vi "Parse MREU Variant.vi"(10 "Variant":variant) -> (2 "MREU Telemetry":T1 {"DSCR"."Raw_DSCR" format="%04x"; "DSCR"."DM_EE_ERRADD"."MSW" format="%02x"; "DSCR"."DM_EE_ERRADD"."LSW" format="%04x"; "DSCR"."DSCR_5"."DM_INTVL" format="%03x"; "DSCR"."TMR_30_31"."TMR1_CNT" format="%1x"; "DSCR"."TMR_30_31"."TMR0_CNT" format="%1x"; "DSCR"."TMR_26_27"."TMR1_CNT" format="%1x"; "DSCR"."TMR_26_27"."TMR0_CNT" format="%1x"; "DSCR"."TMR_24_25"."TMR1_CNT" format="%1x"; "DSCR"."TMR_24_25"."TMR0_CNT" format="%1x"; "DSCR"."TMR_28_29"."TMR1_CNT" format="%1x"; "DSCR"."TMR_28_29"."TMR0_CNT" format="%1x"; "DSCR"."TMR_16_17"."TMR1_CNT" format="%1x"; "DSCR"."TMR_16_17"."TMR0_CNT" format="%1x"; "DSCR"."TMR_22_23"."TMR1_CNT" format="%1x"; "DSCR"."TMR_22_23"."TMR0_CNT" format="%1x"; "DSCR"."TMR_20_21"."TMR1_CNT" format="%1x"; "DSCR"."TMR_20_21"."TMR0_CNT" format="%1x"; "DSCR"."TMR_18_19"."TMR1_CNT" format="%1x"; "DSCR"."TMR_18_19"."TMR0_CNT" format="%1x"; "DSCR"."TMR_14_15"."TMR1_CNT" format="%1x"; "DSCR"."TMR_14_15"."TMR0_CNT" format="%1x"; "DSCR"."TMR_12_13"."TMR1_CNT" format="%1x"; "DSCR"."TMR_12_13"."TMR0_CNT" format="%1x"; "DSCR"."TMR_10_11"."TMR1_CNT" format="%1x"; "DSCR"."TMR_10_11"."TMR0_CNT" format="%1x"; "DSCR"."TMR_8_9"."TMR1_CNT" format="%1x"; "DSCR"."TMR_8_9"."TMR0_CNT" format="%1x"; "DSCR"."TMR_6_7"."TMR1_CNT" format="%1x"; "DSCR"."TMR_6_7"."TMR0_CNT" format="%1x"; "DSCR"."TMR_4_5"."TMR1_CNT" format="%1x"; "DSCR"."TMR_4_5"."TMR0_CNT" format="%1x"; "DSCR"."TMR_2_3"."TMR1_CNT" format="%1x"; "DSCR"."TMR_2_3"."TMR0_CNT" format="%1x"; "DSCR"."TMR_0_1"."TMR1_CNT" format="%1x"; "DSCR"."TMR_0_1"."TMR0_CNT" format="%1x"; "Full ESCR"."RawESCR" format="%04x"; "Full ESCR"."RTR2"."Value" format="%04x"; "Full ESCR"."CLK_DRFT"."Value" format="%04x"; "Full ESCR"."CLK_ADJ"."Value" format="%04x"; "Full ESCR"."MT_ERRADD"."Value" format="%04x"; "Full ESCR"."TC_ERRADD"."Value" format="%04x"; "Full ESCR"."Device_ID"."Value" format="%04x"; "Full ESCR"."SCT"."SCT" format="%04x"; "Full ESCR"."SCT"."RTI" format="%02x"; "Full ESCR"."DMA_ERRADD"."LSW" format="%04x"; "Full ESCR"."DMA_ERRADD"."MSW" format="%02x"; "Full ESCR"."EEPROM_ERRADD"."LSW" format="%04x"; "Full ESCR"."EEPROM_ERRADD"."MSW" format="%02x"; "Full ESCR"."SCR_ERRADD"."LSW" format="%04x"; "Full ESCR"."SCR_ERRADD"."MSW" format="%02x"; "Full_PM"."RawPM" format="%04x"; "Full_PM"."CKSUM"."Value" format="%04x"; "Full_PM"."BUALM_SNZ"."LSW" format="%04x"; "Full_PM"."BUALM_SNZ"."MSW" format="%02x"; "Full_PM"."BUALM"."LSW" format="%04x"; "Full_PM"."BUALM"."MSW" format="%02x"; "Full_PM"."PALM_SNZ"."LSW" format="%04x"; "Full_PM"."PALM_SNZ"."MSW" format="%02x"; "Full_PM"."PALM"."LSW" format="%04x"; "Full_PM"."PALM"."MSW" format="%02x"; "Full_PM"."MissionClock"."Val_19_4" format="%04x"; "Full_PM"."MissionClock"."Val_35_20" format="%04x"; "Full_PM"."MissionClock"."Val_51_36" format="%04x"; "Full_PM"."FP_WDT"."Value" format="%04x"; "Full DISC"."RawDiscIn" format="%04x"; "Full DISC"."RawDISC" format="%04x"})   [LabVIEW 2019]
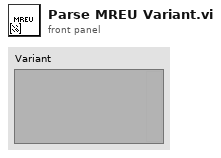
[diagram p1: front panel]
types:
  T1 = cluster{"NoResponse":bool, "Analog Telemetry":waveform(dbl)[], "Full ESCR":cluster{"ESCR 7":cluster{"RT_TC_ERAD_WR":bool, "SCR_ERAD_WR":bool, "EE_ERAD_WR":bool, "DMA_ERAD_WR":bool, "CLKADJ_WR":bool, "CLKDRFT_WR":bool, "MT_ERAD_WR":bool, "BUS_CONF_INH":bool, "VMON_OVRD":bool, "VMN_OVRD_CTL":bool, "PM_TEST_EN":bool, "VMON_P3V":bool, "VMON_P5V":bool, "VMON_N12V":bool, "VMON_P12V":bool, "SET_CLRn":bool}, "ESCR 6":cluster{"DMA_DBE":bool, "DMA_SBE":bool, "UNUSED":bool, "ILL_MEM_ACC":bool, "EE_RD_URUN":bool, "EE_WR_ORUN":bool, "EE_WR_TIMEOUT":bool, "EE_WR_BUSY":bool, "BANK_0_WPV":bool, "BANK_1_WPV":bool, "BANK_2_WPV":bool, "BANK_3_WPV":bool, "FSW_HIMEM_WPV":bool, "FSW_BNK_WPV":bool, "DMA_SRAM_WPV":bool, "SET_CLRn":bool}, "ESCR 5":cluster{"EEPROM_DBE":bool, "EEPROM_SBE":bool, "AI_MOVE_CONF":bool, "DEF_BANK_ERR":bool, "PREEMPTION":bool, "UNEX_OPCODE":bool, "ILLEGAL_OPCOD":bool, "RANGE_ERR":bool, "RSB_ABORT":bool, "TLM_ADDR_CFG":bool, "RZ_EN":bool, "TLM_DATA_ERR":bool, "TLM_TIME_OUT":bool, "TLM_FR_ERR":bool, "TLM_PAR_ERR":bool, "SET_CLRn ":bool}, "ESCR_4":cluster{"ACT_BANK_0":bool, "ACT_BANK_1":bool, "EXT_DEF_BANK_0":bool, "EXT_DEF_BANK_1":bool, "FSW_DEF_BANK_0":bool, "FSW_DEF_BANK_1":bool, "DEF_BANKSEL_0":bool, "DEF_BANKSEL_1":bool, "WP_BNK0_INH":bool, "WP_BNK1_INH":bool, "WP_BNK2_INH":bool, "WP_BNK3_INH":bool, "WP_HIME_INH":bool, "ILL_BNK_CHNG":bool, "WP_SRAM_INH":bool, "SET_CLRn ":bool}, "ESCR 3":cluster{"SCR_DBE":bool, "SCR_SBE":bool, "UNUSED[2]":bool, "UNUSED[3]":bool, "UNUSED[4]":bool, "UNUSED[5]":bool, "SRAM_SCR_EN":bool, "PROM_SCR_EN":bool, "BRG_MOD_0":bool, "BRG_MOD_1":bool, "BRG_MOD_2":bool, "PM_CKSUM_EN":bool, "UNUSED[12]":bool, "UNUSED[13] ":bool, "UNUSED[14]":bool, "SET_CLRn":bool}, "ESCR 2":cluster{"CH_DIS_B":bool, "UNUSED[1]":bool, "LVDS_SCF_B":bool, "RT_SCF_B":bool, "BRG_SCF_B":bool, "BUS_CONF_B":bool, "BR_POW_ON":bool, "BR_POW_EN":bool, "CH_DIS_A":bool, "UNUSED[9]":bool, "LVDS_SCF":bool, "RT_SCF":bool, "BRG_SCF_A":bool, "BUS_CONF_A":bool, "BIDI_EN":bool, "SET_CLRn":bool}, "ESCR 1":cluster{"TC_DBE":bool, "TC_SBE":bool, "RTI_ORUN":bool, "MT_PRG_ERR":bool, "HCR_ERR":bool, "RT_DBE":bool, "RT_SBE":bool, "EDAC_EN":bool, "AZEN":bool, "TC_RUN":bool, "COLD_START":bool, "SSYSF_EXT":bool, "RTI_FREQ_0":bool, "RTI_FREQ_1":bool, "SSYSF_INT":bool, "SET_CLRn":bool}, "CLK_DRFT":cluster{"Value":u16}, "CLK_ADJ":cluster{"Value":u16}, "MT_ERRADD":cluster{"Value":u16}, "TC_ERRADD":cluster{"Value":u16}, "Device_ID":cluster{"Value":u16}, "Board_ID":cluster{"ID":u16, "Board Type":enum16{"BB", "EM_SKT", "EM_AX2K", "EM_RTAX", "FM_SKT", "FM_RTAX"}}, "SCT":cluster{"SCT":u16, "RTI":u8}, "DMA_ERRADD":cluster{"LSW":u16, "MSW":u8}, "EEPROM_ERRADD":cluster{"LSW":u16, "MSW":u8}, "SCR_ERRADD":cluster{"LSW":u16, "MSW":u8}, "RTR2":cluster{"Value":u16}, "RawESCR":u16[]}, "Full_PM":cluster{"CKSUM":cluster{"Value":u16}, "PWR_LDSHD":cluster{"LOADSHED_PWR_L":bool, "LOADSHED_PWR_H":bool, "UNUSED[2]":bool, "UNUSED[3]":bool, "UNUSED[4]":bool, "UNUSED[5]":bool, "UNUSED[6]":bool, "UNUSED[7]":bool, "LOADSHEDL_EN":bool, "LOADSHEDH_EN":bool, "XSWU_OUT_MSK":bool, "UNUSED[11]":bool, "UNUSED[12]":bool, "UNUSED[13]":bool, "UNUSED[14]":bool, "SET_CLRn":bool}, "FPWDG_STAT":cluster{"UNUSED[0]":bool, "UNUSED[1]":bool, "UNUSED[2]":bool, "UNUSED[3]":bool, "UNUSED[4]":bool, "UNUSED[5]":bool, "UNUSED[6]":bool, "UNUSED[7]":bool, "UNUSED[8]":bool, "UNUSED[9]":bool, "FPWDG_INH":bool, "FPWDG_INH0":bool, "FPWDG_INH1":bool, "FPWDG_INH2":bool, "FPWDG_EXP":bool, "UNUSED[15]":bool}, "PWR_STAT":cluster{"POR1_EVT":bool, "POR2_EVT":bool, "PALM_EXP_EVT":bool, "XSWU_IN_EVT":bool, "USER1_EVT":bool, "USER2_EVT":bool, "GSE_EVT":bool, "POWER_POS_EVT":bool, "BOI_EVT":bool, "BUALM_EXP_EVT":bool, "UV_TRIP_EVT":bool, "MCLOCK_0":bool, "MCLOCK_1":bool, "MCLOCK_2":bool, "MCLOCK_3":bool, "SET_CLRn":bool}, "PWR_MSK":cluster{"UNUSED[0]":bool, "POR2_MSK":bool, "PALM_EXP_MSK":bool, "XSWU_IN_MSK":bool, "USER1_MSK":bool, "USER2_MSK":bool, "GSE_MSK":bool, "PWR_POS_MSK":bool, "BOI_MSK":bool, "BUALM_EXP_MSK":bool, "UV_TRIP_MSK":bool, "UNUSED[11]":bool, "BUALM_STEER":bool, "SELFCHK_MSK":bool, "CHKSUM_FAIL":bool, "SET_CLRn":bool}, "PWR_ACK":cluster{"COLD_START":bool, "POR2_WU":bool, "PALM_EXP_WU":bool, "XSWU_IN_WU":bool, "USER1_WU":bool, "USER2_WU":bool, "GSE_WU":bool, "POWER_POS_WU":bool, "BOI":bool, "BUALM_EXP":bool, "UV_TRIP":bool, "NAPPED":bool, "BUALM_EXP_WU":bool, "SELFCHK_FAIL":bool, "SLEEP_PNDG":bool, "SET_CLRn":bool}, "PWR_CTRL":cluster{"PWR_EN":bool, "PALM_VALID":bool, "PALM_SNZ_VALID":bool, "BUALM_VALID":bool, "BUALM_SNZ_VALID":bool, "MC_VALID":bool, "UNUSED[6]":bool, "FSM_BIT":bool, "Prev_State":enum16{"Sleep_00", "Deadman_01", "Awake_10", "Nap_11"}, "Curr_State":enum16{"Sleep_00", "Deadman_01", "Awake_10", "Nap_11"}, "POWER_POS":bool, "UNUSED[13]":bool, "UNUSED[14]":bool, "SET_CLRn":bool}, "BUALM_SNZ":cluster{"LSW":u16, "MSW":u8}, "BUALM":cluster{"LSW":u16, "MSW":u8}, "PALM_SNZ":cluster{"LSW":u16, "MSW":u8}, "PALM":cluster{"LSW":u16, "MSW":u8}, "MissionClock":cluster{"Val_19_4":u16, "Val_35_20":u16, "Val_51_36":u16}, "FP_WDT":cluster{"Value":u16}, "PWR_OFF_EN":cluster{"PWR_OFF_L_0":bool, "PWR_OFF_H_0":bool, "PWR_OFF_L_1":bool, "PWR_OFF_H_1":bool, "PWR_OFF_L_2":bool, "PWR_OFF_H_2":bool, "PWR_OFF_L_3":bool, "PWR_OFF_H_3":bool, "PWR_OFF_L_4":bool, "PWR_OFF_H_4":bool, "PWR_OFF_L_5":bool, "PWR_OFF_H_5":bool, "PWR_OFF_L_6":bool, "PWR_OFF_H_6":bool, "UNUSED[14]":bool, "SET_CLRn":bool}, "PWR_ON_EN":cluster{"PWR_ON_L_0":bool, "PWR_ON_H_0":bool, "PWR_ON_L_1":bool, "PWR_ON_H_1":bool, "PWR_ON_L_2":bool, "PWR_ON_H_2":bool, "PWR_ON_L_3":bool, "PWR_ON_H_3":bool, "PWR_ON_L_4":bool, "PWR_ON_H_4":bool, "PWR_ON_L_5":bool, "PWR_ON_H_5":bool, "PWR_ON_L_6":bool, "PWR_ON_H_6":bool, "UNUSED[14]":bool, "SET_CLRn":bool}, "PWR_PAROUT":cluster{"USER0_PWR_L":bool, "USER0_PWR_H":bool, "USER1_PWR_L":bool, "USER1_PWR_H":bool, "USER2_PWR_L":bool, "USER2_PWR_H":bool, "USER3_PWR_L":bool, "USER3_PWR_H":bool, "USER4_PWR_L":bool, "USER4_PWR_H":bool, "USER5_PWR_L":bool, "USER5_PWR_H":bool, "USER6_PWR_L":bool, "USER6_PWR_H":bool, "UNUSED[14]":bool, "SET_CLRn":bool}, "PWR_PANIC_EN":cluster{"PWR_PANIC_L_0":bool, "PWR_PANIC_H_0":bool, "PWR_PANIC_L_1":bool, "PWR_PANIC_H_1":bool, "PWR_PANIC_L_2":bool, "PWR_PANIC_H_2":bool, "PWR_PANIC_L_3":bool, "PWR_PANIC_H_3":bool, "PWR_PANIC_L_4":bool, "PWR_PANIC_H_4":bool, "PWR_PANIC_L_5":bool, "PWR_PANIC_H_5":bool, "PWR_PANIC_L_6":bool, "PWR_PANIC_H_6":bool, "UNUSED[14]":bool, "SET_CLRn":bool}, "RawPM":u16[]}, "Full DISC":cluster{"Discrete_Status":cluster{"STAT_0":bool, "STAT_1":bool, "STAT_2":bool, "STAT_3":bool, "STAT_4":bool, "STAT_5":bool, "STAT_6":bool, "STAT_7":bool}, "Discrete_Out":cluster{"DISC_RST":bool, "DISCO_1":bool, "DISCO_2":bool, "DISCO_3":bool, "DISCO_4":bool, "DISCO_5":bool, "DISCO_6":bool, "DISCO_7":bool}, "Discrete_Settings":cluster{"WP_DIS_WR":bool, "WDT_DIS_WR":bool, "WPV_WR":bool, "WDT_XPIRD_WR":bool, "WP_DIS":bool, "WPV":bool, "WDT_DIS":bool, "WDT_XPIRD":bool}, "Discrete In":cluster{"DISC_IN_00":bool, "DISC_IN_01":bool, "DISC_IN_02":bool, "DISC_IN_03":bool, "DISC_IN_04":bool, "DISC_IN_05":bool, "DISC_IN_06":bool, "DISC_IN_07":bool, "DISC_IN_08":bool, "DISC_IN_09":bool, "DISC_IN_10":bool, "DISC_IN_11":bool, "DISC_IN_12":bool, "DISC_IN_13":bool, "DISC_IN_14":bool, "DISC_IN_15":bool}, "Test_Enabled":bool, "DISCO_Reset":bool, "WDT":u8, "RawDISC":u16[], "RawDiscIn":u16}, "DSCR":cluster{"DSCR_1":cluster{"MCT_NENTRY":u8, "Spare":u8, "TIMRSTAT_CLR":bool, "MCT_VALID":bool, "EXPTIME_VALID":bool, "INTVL_VALID":bool, "ERRADD_VALID":bool, "RUNNING":bool, "DM_EN":bool, "SET_CLRn":bool}, "DSCR_2":cluster{"DM_DBE":bool, "DM_SBE":bool, "DM_MT_WPV":bool, "DM_MT_PROGERR":bool, "SPARE_4":bool, "DM_UEOPER":bool, "DM_ILLOPERR":bool, "DM_RNGERR":bool, "DM_PERIOD_ERR":bool, "DM_RSB_ADDRCONF":bool, "DM_CSUMERR":bool, "DM_RSB_DATAERR":bool, "DM_RSB_TIMEOUT":bool, "DM_RSB_FRMERR":bool, "DM_RSB_PARERR":bool, "SET_CLRn":bool}, "DSCR_3":cluster{"MCT_BASE_ADDR":u16}, "DSCR_4":cluster{"DM_EXPTIME":u16}, "DSCR_5":cluster{"DM_INTVL":u16}, "DM_EE_ERRADD":cluster{"MSW":u16, "LSW":u16}, "TMR_0_1":cluster{"TMR0_CNT":u8, "TMR0_CNT_OVFL":bool, "TMR0_TYPE":enum8{"No-Op", "Absolute", "Periodic", "Hybrid"}, "TMR0_EX":bool, "TMR1_CNT":u8, "TMR1_CNT_OVFL":bool, "TMR1_TYPE":enum8{"No-Op", "Absolute", "Periodic", "Hybrid"}, "TMR1_EX":bool}, "TMR_2_3":cluster{"TMR0_CNT":u8, "TMR0_CNT_OVFL":bool, "TMR0_TYPE":enum8{"No-Op", "Absolute", "Periodic", "Hybrid"}, "TMR0_EX":bool, "TMR1_CNT":u8, "TMR1_CNT_OVFL":bool, "TMR1_TYPE":enum8{"No-Op", "Absolute", "Periodic", "Hybrid"}, "TMR1_EX":bool}, "TMR_4_5":cluster{"TMR0_CNT":u8, "TMR0_CNT_OVFL":bool, "TMR0_TYPE":enum8{"No-Op", "Absolute", "Periodic", "Hybrid"}, "TMR0_EX":bool, "TMR1_CNT":u8, "TMR1_CNT_OVFL":bool, "TMR1_TYPE":enum8{"No-Op", "Absolute", "Periodic", "Hybrid"}, "TMR1_EX":bool}, "TMR_6_7":cluster{"TMR0_CNT":u8, "TMR0_CNT_OVFL":bool, "TMR0_TYPE":enum8{"No-Op", "Absolute", "Periodic", "Hybrid"}, "TMR0_EX":bool, "TMR1_CNT":u8, "TMR1_CNT_OVFL":bool, "TMR1_TYPE":enum8{"No-Op", "Absolute", "Periodic", "Hybrid"}, "TMR1_EX":bool}, "TMR_8_9":cluster{"TMR0_CNT":u8, "TMR0_CNT_OVFL":bool, "TMR0_TYPE":enum8{"No-Op", "Absolute", "Periodic", "Hybrid"}, "TMR0_EX":bool, "TMR1_CNT":u8, "TMR1_CNT_OVFL":bool, "TMR1_TYPE":enum8{"No-Op", "Absolute", "Periodic", "Hybrid"}, "TMR1_EX":bool}, "TMR_10_11":cluster{"TMR0_CNT":u8, "TMR0_CNT_OVFL":bool, "TMR0_TYPE":enum8{"No-Op", "Absolute", "Periodic", "Hybrid"}, "TMR0_EX":bool, "TMR1_CNT":u8, "TMR1_CNT_OVFL":bool, "TMR1_TYPE":enum8{"No-Op", "Absolute", "Periodic", "Hybrid"}, "TMR1_EX":bool}, "TMR_12_13":cluster{"TMR0_CNT":u8, "TMR0_CNT_OVFL":bool, "TMR0_TYPE":enum8{"No-Op", "Absolute", "Periodic", "Hybrid"}, "TMR0_EX":bool, "TMR1_CNT":u8, "TMR1_CNT_OVFL":bool, "TMR1_TYPE":enum8{"No-Op", "Absolute", "Periodic", "Hybrid"}, "TMR1_EX":bool}, "TMR_14_15":cluster{"TMR0_CNT":u8, "TMR0_CNT_OVFL":bool, "TMR0_TYPE":enum8{"No-Op", "Absolute", "Periodic", "Hybrid"}, "TMR0_EX":bool, "TMR1_CNT":u8, "TMR1_CNT_OVFL":bool, "TMR1_TYPE":enum8{"No-Op", "Absolute", "Periodic", "Hybrid"}, "TMR1_EX":bool}, "TMR_16_17":cluster{"TMR0_CNT":u8, "TMR0_CNT_OVFL":bool, "TMR0_TYPE":enum8{"No-Op", "Absolute", "Periodic", "Hybrid"}, "TMR0_EX":bool, "TMR1_CNT":u8, "TMR1_CNT_OVFL":bool, "TMR1_TYPE":enum8{"No-Op", "Absolute", "Periodic", "Hybrid"}, "TMR1_EX":bool}, "TMR_18_19":cluster{"TMR0_CNT":u8, "TMR0_CNT_OVFL":bool, "TMR0_TYPE":enum8{"No-Op", "Absolute", "Periodic", "Hybrid"}, "TMR0_EX":bool, "TMR1_CNT":u8, "TMR1_CNT_OVFL":bool, "TMR1_TYPE":enum8{"No-Op", "Absolute", "Periodic", "Hybrid"}, "TMR1_EX":bool}, "TMR_20_21":cluster{"TMR0_CNT":u8, "TMR0_CNT_OVFL":bool, "TMR0_TYPE":enum8{"No-Op", "Absolute", "Periodic", "Hybrid"}, "TMR0_EX":bool, "TMR1_CNT":u8, "TMR1_CNT_OVFL":bool, "TMR1_TYPE":enum8{"No-Op", "Absolute", "Periodic", "Hybrid"}, "TMR1_EX":bool}, "TMR_22_23":cluster{"TMR0_CNT":u8, "TMR0_CNT_OVFL":bool, "TMR0_TYPE":enum8{"No-Op", "Absolute", "Periodic", "Hybrid"}, "TMR0_EX":bool, "TMR1_CNT":u8, "TMR1_CNT_OVFL":bool, "TMR1_TYPE":enum8{"No-Op", "Absolute", "Periodic", "Hybrid"}, "TMR1_EX":bool}, "TMR_24_25":cluster{"TMR0_CNT":u8, "TMR0_CNT_OVFL":bool, "TMR0_TYPE":enum8{"No-Op", "Absolute", "Periodic", "Hybrid"}, "TMR0_EX":bool, "TMR1_CNT":u8, "TMR1_CNT_OVFL":bool, "TMR1_TYPE":enum8{"No-Op", "Absolute", "Periodic", "Hybrid"}, "TMR1_EX":bool}, "TMR_26_27":cluster{"TMR0_CNT":u8, "TMR0_CNT_OVFL":bool, "TMR0_TYPE":enum8{"No-Op", "Absolute", "Periodic", "Hybrid"}, "TMR0_EX":bool, "TMR1_CNT":u8, "TMR1_CNT_OVFL":bool, "TMR1_TYPE":enum8{"No-Op", "Absolute", "Periodic", "Hybrid"}, "TMR1_EX":bool}, "TMR_28_29":cluster{"TMR0_CNT":u8, "TMR0_CNT_OVFL":bool, "TMR0_TYPE":enum8{"No-Op", "Absolute", "Periodic", "Hybrid"}, "TMR0_EX":bool, "TMR1_CNT":u8, "TMR1_CNT_OVFL":bool, "TMR1_TYPE":enum8{"No-Op", "Absolute", "Periodic", "Hybrid"}, "TMR1_EX":bool}, "TMR_30_31":cluster{"TMR0_CNT":u8, "TMR0_CNT_OVFL":bool, "TMR0_TYPE":enum8{"No-Op", "Absolute", "Periodic", "Hybrid"}, "TMR0_EX":bool, "TMR1_CNT":u8, "TMR1_CNT_OVFL":bool, "TMR1_TYPE":enum8{"No-Op", "Absolute", "Periodic", "Hybrid"}, "TMR1_EX":bool}, "Raw_DSCR":u16[]}}
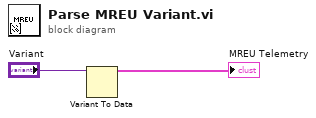
[diagram p0: block diagram]
diagram:
  n1 = Variant To Data(Variant="Variant") -> (data=→"MREU Telemetry":T1)  [unwired: 2 in, 1 out]
